vi "DamnYankeeHindbrainRemoteControlSense.vi"(10 "Notifier References":T9, 11 "IO Cluster":T1) -> (0 "Error out":errorcluster)   [LabVIEW 2013]
doc: "This VI reads the remote control data that is coming in and continually updates what the boat thinks the controller is doing. It's in a separate while loop from the rest of the Sense data because the direct reading of PWM signals requires a somewhat consistent time-step.\n\nEric Schneider, May 2014"
uses:
  Data/TypeDefs/Notifiers.ctl
  Data/TypeDefs/UTM Location.ctl
  Data/TypeDefs/Sail Set Suggestions.ctl
  Data/TypeDefs/Rudder Set Suggestions.ctl
  Data/TypeDefs/OverrideInformation.ctl
  Data/TypeDefs/OverrideMode.ctl
  Data/TypeDefs/MotorSetup.ctl
  Data/TypeDefs/DynamixelSetupInfo.ctl
  Data/TypeDefs/AirmarStatus.ctl
  Data/TypeDefs/HardwareOnline.ctl
  Data/TypeDefs/DynamixelCycleTracker.ctl
  Data/TypeDefs/RC Input Values.ctl
  Data/TypeDefs/DamnYankeeIOPorts.ctl
  <vilib>/myRIO/Instrument Drivers/Onboard IO/DIO/typedefs/DIO Reference.ctl
  <vilib>/myRIO/Common/Instrument Driver Framework/Utilities/typedefs/myRIO Generic Hardware Reference.ctl
  <vilib>/myRIO/Common/Instrument Driver Framework/Utilities/typedefs/Hardware Version Enum.ctl
  <vilib>/myRIO/Common/Instrument Driver Framework/Utilities/typedefs/myRIO v1.0 Reference.ctl
  <vilib>/myRIO/Common/Instrument Driver Framework/Utilities/typedefs/Generic FPGA Reference.ctl
  <vilib>/myRIO/Common/Instrument Driver Framework/myRIO v1.0/DIO/typedefs/DIO Channels List.ctl
  <vilib>/myRIO/Common/Instrument Driver Framework/myRIO v1.0/DIO/typedefs/DIO Channels Enum.ctl
  <vilib>/Utility/error.llb/Error Cluster From Error Code.vi
  <vilib>/myRIO/Common/Instrument Driver Framework/myRIO v1.0/DIO/vis/myRIO v1.0 Read DIO.vi
  <vilib>/myRIO/Instrument Drivers/Onboard IO/DIO/DIO.lvlib
panel:
  out "Switch value":dbl
  out "Sail value":dbl
  out "Rudder value":dbl
  # "Debugging information"
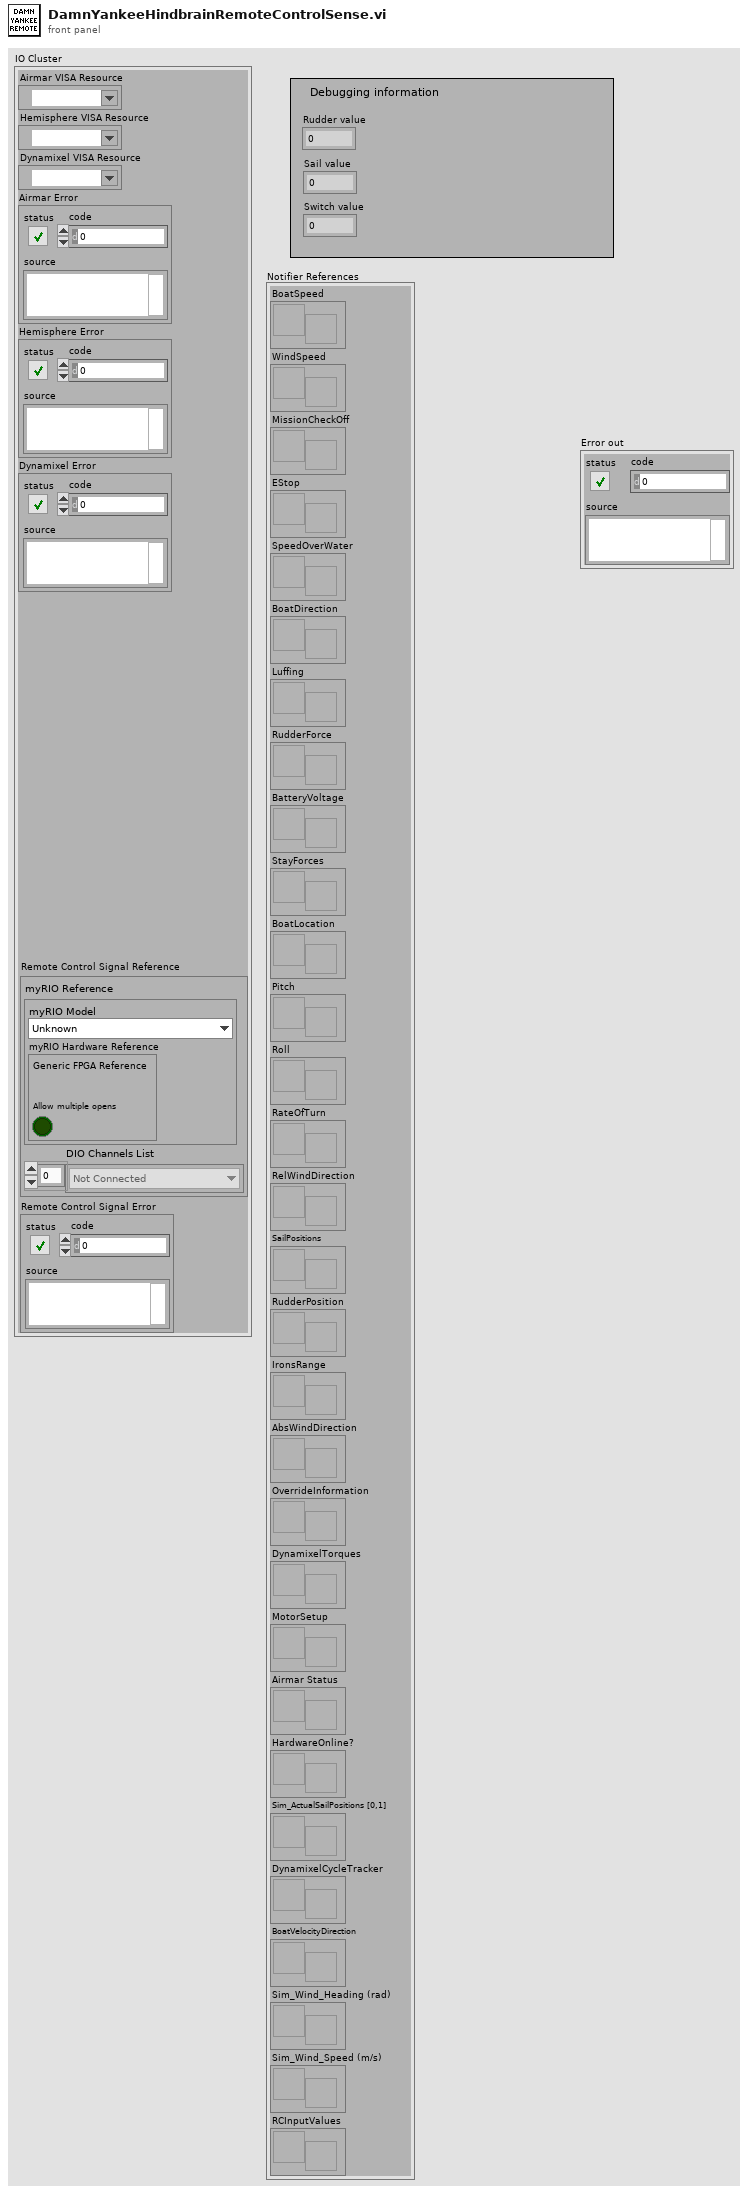
[diagram p1: front panel]
types:
  T1 = typedef "DamnYankeeIOPorts.ctl" = cluster{"Airmar VISA Resource":refnum<visa-resource-name>, "Hemisphere VISA Resource":refnum<visa-resource-name>, "Dynamixel VISA Resource":refnum<visa-resource-name>, "Airmar Error":errorcluster, "Hemisphere Error":errorcluster, "Dynamixel Error":errorcluster, "Remote Control Signal Reference":T2, "Remote Control Signal Error":errorcluster}
  T2 = typedef "DIO.lvlib/DIO Reference.ctl" = cluster{"myRIO Reference":T3, "DIO Channels List":T7}
  T3 = typedef "myRIO Generic Hardware Reference.ctl" = cluster{"myRIO Model":T4, "myRIO Hardware Reference":T5}
  T4 = typedef "Hardware Version Enum.ctl" = enum16{"Unknown", "myRIO-1900", "myRIO-1950"}
  T5 = typedef "myRIO v1.0 Reference.ctl" = cluster{"Generic FPGA Reference":T6, "Allow multiple opens":bool}
  T6 = typedef "Generic FPGA Reference.ctl" = refnum<k20>
  T7 = typedef "DIO Channels List.ctl" = T8[]
  T8 = typedef "DIO Channels Enum.ctl" = enum16{"Not Connected", "C/DIO0", "C/DIO1", "C/DIO2", "C/DIO3", "C/DIO4", "C/DIO5", "C/DIO6", "C/DIO7", "A/DIO0", "A/DIO1", "A/DIO2", "A/DIO3", "A/DIO4", "A/DIO5", "A/DIO6", "A/DIO7", "A/DIO8", "A/DIO9", "A/DIO10", "A/DIO11", "A/DIO12", "A/DIO13", "A/DIO14", "A/DIO15", "B/DIO0", "B/DIO1", "B/DIO2", "B/DIO3", "B/DIO4", "B/DIO5", "B/DIO6", "B/DIO7", "B/DIO8", "B/DIO9", "B/DIO10", "B/DIO11", "B/DIO12", "B/DIO13", "B/DIO14", "B/DIO15", "LED0", "LED1", "LED2", "LED3", "Button0"}
  T9 = typedef "Notifiers.ctl" = cluster{"BoatSpeed":refnum<notifier>, "WindSpeed":refnum<notifier>, "MissionCheckOff":refnum<notifier>, "EStop":refnum<notifier>, "SpeedOverWater":refnum<notifier>, "BoatDirection":refnum<notifier>, "Luffing":refnum<notifier>, "RudderForce":refnum<notifier>, "BatteryVoltage":refnum<notifier>, "StayForces":refnum<notifier>, "BoatLocation":refnum<notifier>, "Pitch":refnum<notifier>, "Roll":refnum<notifier>, "RateOfTurn":refnum<notifier>, "RelWindDirection":refnum<notifier>, "SailPositions":refnum<notifier>, "RudderPosition":refnum<notifier>, "IronsRange":refnum<notifier>, "AbsWindDirection":refnum<notifier>, "OverrideInformation":refnum<notifier>, "DynamixelTorques":refnum<notifier>, "MotorSetup":refnum<notifier>, "Airmar Status":refnum<notifier>, "HardwareOnline?":refnum<notifier>, "Sim_ActualSailPositions [0,1]":refnum<notifier>, "DynamixelCycleTracker":refnum<notifier>, "BoatVelocityDirection":refnum<notifier>, "Sim_Wind_Heading (rad)":refnum<notifier>, "Sim_Wind_Speed (m/s)":refnum<notifier>, "RCInputValues":refnum<notifier>}
  T10 = typedef "RC Input Values.ctl" = cluster{"RC Switch Value":dbl, "Sail setpoints":T11, "Rudder Setpoint":T12}
  T11 = typedef "Sail Set Suggestions.ctl" = cluster{"MainSailSuggestion":dbl, "JibSailSuggestion":dbl}
  T12 = typedef "Rudder Set Suggestions.ctl" = dbl
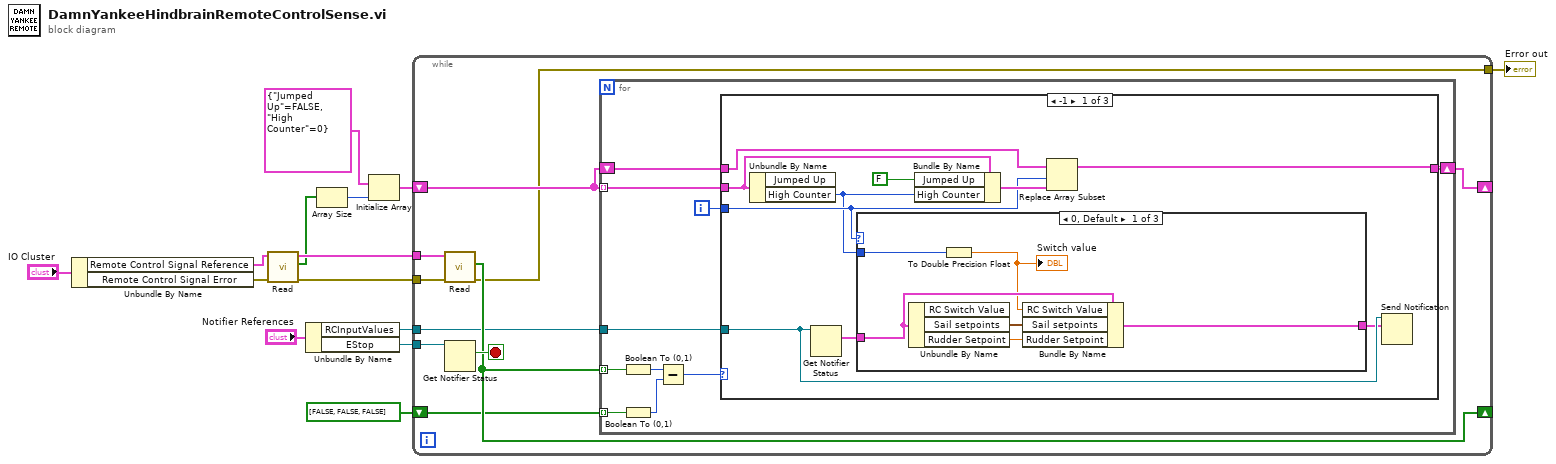
[diagram p0: block diagram]
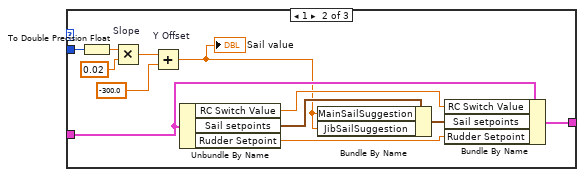
[diagram p2: hidden frame]
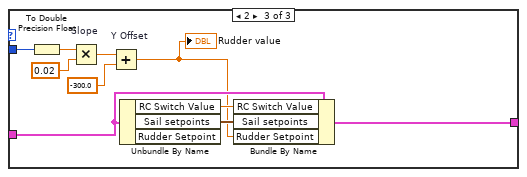
[diagram p3: hidden frame]
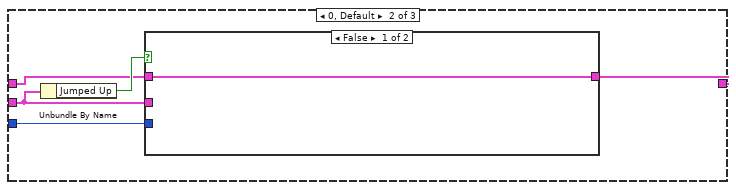
[diagram p4: hidden frame]
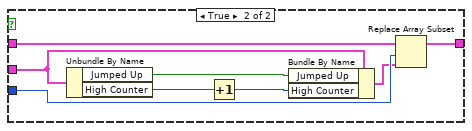
[diagram p5: hidden frame]
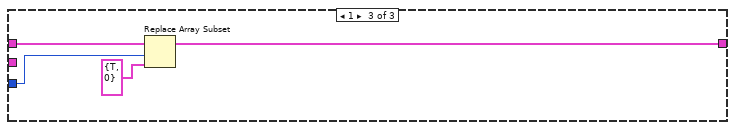
[diagram p6: hidden frame]
diagram:
  n1 = Unbundle By Name("IO Cluster") -> ("Remote Control Signal Reference"=w7:T2, "Remote Control Signal Error"=w6:errorcluster)
  n2 = call <vilib>:"Read.vi"("error in (no error)"=w6, "DIO Ref In"=w7) -> ("error out"=w4:errorcluster, "Values"=w3:bool[], "DIO Ref Out"=w5:T2)  [unwired: 7 in]
  n3 = Unbundle By Name("Notifier References") -> ("RCInputValues"=w12:refnum<notifier>, "EStop"=w11:refnum<notifier>)
  n4 = Array Size(array=w3) -> (size(s)=w2:i32)
  n5 = Initialize Array(cluster{"Jumped Up":bool, "High Counter":i32} {"Jumped Up"=FALSE, "High Counter"=0}, w2) -> (w9:cluster{"Jumped Up":bool, "High Counter":i32}[])
  n6 = while {
    tunnel: w11 -> [w24]
    tunnel: w12 -> [w16]
    tunnel: w5 -> [w22]
    tunnel: w4 -> [w21]
    shift-right: [w20] -> _
    shift-left: bool[] [FALSE, FALSE, FALSE] ("Values") -> [w19]
    shift-right: [w17] -> _
    shift-left: w9 -> [w18]
    tunnel: [w15] -> w1
    stop <- w23 stop-if-true
    n7 = call <vilib>:"Read.vi"("error in (no error)"=w21, "DIO Ref In"=w22) -> ("error out"=w15:errorcluster, "Values"=w20:bool[])  [unwired: 7 in, 1 out]
    n8 = Get Notifier Status(notifier=w24) -> (current notification=w23:bool)  [unwired: 1 in, 4 out]
    n9 = for {
      tunnel: w20 -> [w33] mode=indexing
      tunnel: w19 -> [w34] mode=indexing
      tunnel: w18 -> [w29] mode=indexing
      shift-right: [w26] -> w17
      shift-left: w18 -> [w28]
      tunnel: w16 -> [w25]
      i -> [w27]
      n10 = Boolean To (0,1)(Boolean=w33) -> (0, 1=w31:i16)
      n11 = Boolean To (0,1)(Boolean=w34) -> (0, 1=w30:i16)
      n12 = Subtract(x=w31, y=w30) -> (x-y=w32:i16)
      n13 = case shown="-1" w32 {
        tunnel: w29 -> [w42 w76 _]
        tunnel: w28 -> [w43 w75 w90]
        tunnel: w27 -> [w39 w74 w89]
        tunnel: [w40 w73 w88] -> w26
        tunnel: w25 -> [w37 _ _]
        frame -1 {
          n14 = Unbundle By Name(w42) -> ("High Counter"=w35:i32)  [unwired: 1 out]
          n15 = Get Notifier Status(notifier=w37) -> (current notification=w38:T10)  [unwired: 1 in, 4 out]
          n16 = case shown="0, Default" w39 {
            tunnel: w38 -> [w48 w60 w70]
            tunnel: [w47 w59 w69] -> w36
            tunnel: w35 -> [w46 w51 w68]
            frame 0, Default {
              n17 = Unbundle By Name(w48) -> ("Sail setpoints"=w50:T11, "Rudder Setpoint"=w49:T12)  [unwired: 1 out]
              n18 = To Double Precision Float(number=w46) -> (double precision float=w45:dbl)
              "Switch value" <- w45
              n19 = Bundle By Name(cluster=w48, "RC Switch Value"=w45, "Sail setpoints"=w50, "Rudder Setpoint"=w49) -> (w47:T10)
            }
            frame 1 {
              n20 = To Double Precision Float(number=w51) -> (double precision float=w56:dbl)
              n21 = Multiply "Slope"(x=w56, y=0.02) -> (x*y=w54:dbl)
              n22 = Add "Y Offset"(x=w54, y=-300.0) -> (x+y=w52:dbl)
              "Sail value" <- w52
              n23 = Unbundle By Name(w60) -> ("RC Switch Value"=w62:dbl, "Sail setpoints"=w58:T11, "Rudder Setpoint"=w61:T12)
              n24 = Bundle By Name(cluster=w58, "MainSailSuggestion"=w52, "JibSailSuggestion"=w52) -> (w57:T11)
              n25 = Bundle By Name(cluster=w60, "RC Switch Value"=w62, "Sail setpoints"=w57, "Rudder Setpoint"=w61) -> (w59:T10)
            }
            frame 2 {
              n26 = To Double Precision Float(number=w68) -> (double precision float=w67:dbl)
              n27 = Multiply "Slope"(x=w67, y=0.02) -> (x*y=w65:dbl)
              n28 = Add "Y Offset"(x=w65, y=-300.0) -> (x+y=w63:dbl)
              "Rudder value" <- w63
              n29 = Unbundle By Name(w70) -> ("RC Switch Value"=w71:dbl, "Sail setpoints"=w72:T11)  [unwired: 1 out]
              n30 = Bundle By Name(cluster=w70, "RC Switch Value"=w71, "Sail setpoints"=w72, "Rudder Setpoint"=w63) -> (w69:T10)
            }
          }
          n31 = Bundle By Name(cluster=w42, "Jumped Up"=FALSE, "High Counter"=w35) -> (w44:cluster{"Jumped Up":bool, "High Counter":i32})
          n32 = Replace Array Subset(array=w43, new element=w44, index=w39) -> (w40:cluster{"Jumped Up":bool, "High Counter":i32}[])
          n33 = Send Notification(notification=w36, notifier=w37) -> ()  [unwired: 1 in, 2 out]
        }
        frame 0, Default {
          n34 = Unbundle By Name(w76) -> ("Jumped Up"=w77:bool)
          n35 = case shown="False" w77 {
            tunnel: w76 -> [_ w86]
            tunnel: w75 -> [w78 w82]
            tunnel: w74 -> [_ w81]
            tunnel: [w78 w79] -> w73
            frame False {
            }
            frame True {
              n36 = Unbundle By Name(w86) -> ("Jumped Up"=w85:bool, "High Counter"=w84:i32)
              n37 = Increment(x=w84) -> (x+1=w83:i32)
              n38 = Bundle By Name(cluster=w86, "Jumped Up"=w85, "High Counter"=w83) -> (w80:cluster{"Jumped Up":bool, "High Counter":i32})
              n39 = Replace Array Subset(array=w82, new element=w80, index=w81) -> (w79:cluster{"Jumped Up":bool, "High Counter":i32}[])
            }
          }
        }
        frame 1 {
          n40 = Replace Array Subset(array=w90, new element=cluster{"Jumped Up":bool, "High Counter":i32} {"Jumped Up"=TRUE, "High Counter"=0} ("new element/subarray"), index=w89) -> (w88:cluster{"Jumped Up":bool, "High Counter":i32}[])
        }
      }
    }
  }
  "Error out" <- w1
